vi "GFITS_LibSetNmemBufs.vi"(8 "error in (no error)":errorcluster, 10 "numbufs":i16) -> (0 "error out":errorcluster, 2 "return value":i32)   [LabVIEW 2016]
uses:
  c/lib/libgfits.so
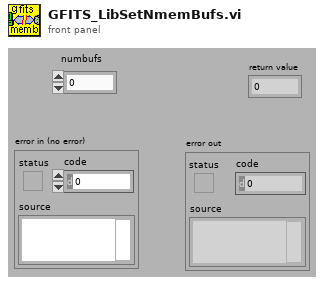
[diagram p1: front panel]
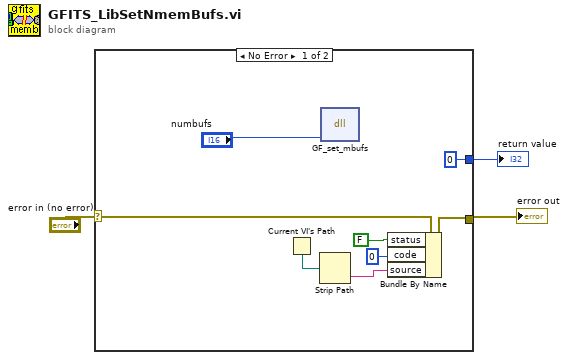
[diagram p0: block diagram]
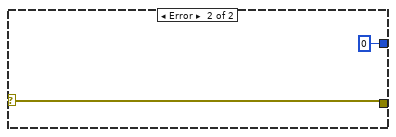
[diagram p2: hidden frame]
diagram:
  n1 = case shown="No Error" "error in (no error)" {
    selector: "error in (no error)" -> [w11 w13]
    tunnel: [0 0] -> w3
    tunnel: [w8 w13] -> w1
    frame No Error {
      n2 = Current VI's Path() -> (path=w10:path)
      n3 = Strip Path(path=w10) -> (name=w9:string)  [unwired: 1 out]
      n4 = dll-call lib="home/simager/panview/PAN/Modules/GFITS/private/c/lib/libgfits.so" fn="GF_set_mbufs"("mbufs"="numbufs") -> ()  [unwired: 4 in, 3 out]
      n5 = Bundle By Name(cluster=w11, "status"=FALSE, "code"=0, "source"=w9) -> (w8:errorcluster)
    }
    frame Error {
    }
  }
  "return value" <- w3
  "error out" <- w1
